vi "PlayWithSync.vi"() -> ()   [LabVIEW 2017]
uses:
  <vilib>/DAQmx/write.llb/DAQmx Write (Digital Wfm 1Chan NSamp).vi
  <vilib>/DAQmx/write.llb/DAQmx Write (Analog 1D Wfm NChan NSamp).vi
  <vilib>/DAQmx/create/channels.llb/DAQmx Create Channel (AO-Voltage-Basic).vi
  <vilib>/DAQmx/create/channels.llb/DAQmx Create Channel (DO-Digital Output).vi
  <vilib>/Waveform/DWDTOps.llb/DWDT Analog to Digital.vi
  <vilib>/DAQmx/configure/timing.llb/DAQmx Timing (Use Waveform).vi
  <vilib>/DAQmx/miscellaneous.llb/DAQmx Fill In Error Info.vi
  <vilib>/Waveform/DWDTOps.llb/DWDT Uncompress Digital.vi
panel:
  in  "Analog Input Sample Clock Source":tag="/Dev1/ao/SampleClock"
  in  "4k Hz Filter":bool=TRUE
  in  "Line(s)":tag="Dev1/port0/line0"
  in  "Physical Channels":tag="Dev1/ao0:1"
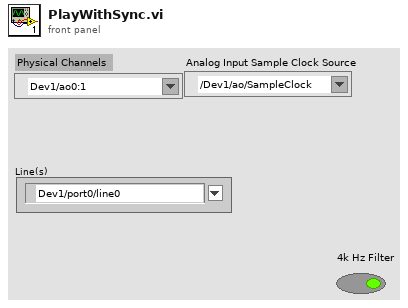
[diagram p1: front panel]
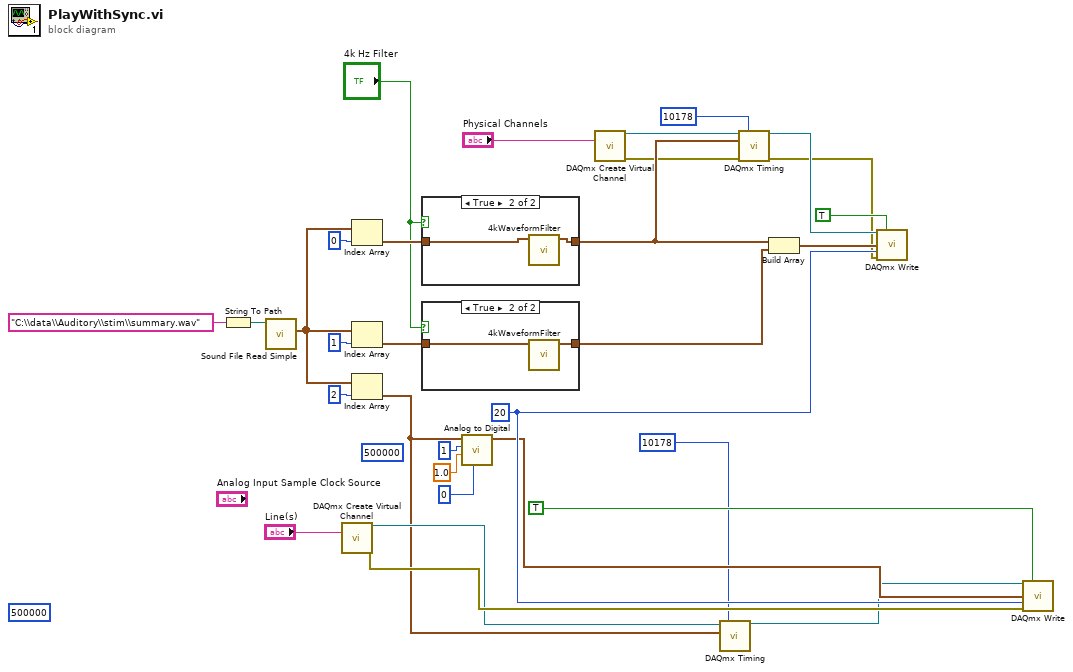
[diagram p0: block diagram]
diagram:
  (unwired) 500000
  (unwired) 500000
  w15 = 20
  n1 = String To Path(string="C:\\data\\Auditory\\stim\\summary.wav") -> (path=w31:path)
  n2 = call <vilib>:"Sound File Read Simple.vi"("path"=w31) -> ("data"=w25:waveform(dbl)[])  [unwired: 7 in, 3 out]
  n3 = call-poly <vilib>:"DAQmx Create Virtual Channel.vi"("lines"="Line(s)") -> ("task out"=w5:refnum<k21>, "error out"=w7:errorcluster)  [unwired: 13 in]
  n4 = Index Array(array=w25, index=0) -> (element=w18:waveform(dbl))
  n5 = Index Array(array=w25, index=1) -> (element=w19:waveform(dbl))
  n6 = Index Array(array=w25, index=2) -> (element=w2:waveform(dbl))
  n7 = case shown="True" "4k Hz Filter" {
    tunnel: w18 -> [w32 w34]
    tunnel: [w32 w33] -> w11
    frame False {
    }
    frame True {
      n8 = call "4kWaveformFilter.vi"("data"=w34) -> ("Waveform"=w33:waveform(dbl))  [unwired: 10 in]
    }
  }
  n9 = case shown="True" "4k Hz Filter" {
    tunnel: w19 -> [w35 w37]
    tunnel: [w35 w36] -> w14
    frame False {
    }
    frame True {
      n10 = call "4kWaveformFilter.vi"("data"=w37) -> ("Waveform"=w36:waveform(dbl))  [unwired: 10 in]
    }
  }
  n11 = call-poly <vilib>:"Analog to Digital.vi"("data format (offset binary)"=0, "full-scale range (pk-pk)"=1.0, "resolution (16 bit)"=1, "analog waveform"=w2) -> ("digital waveform"=w6:digitalwaveform)  [unwired: 4 in, 3 out]
  n12 = call-poly <vilib>:"DAQmx Create Virtual Channel.vi"("physical channels"="Physical Channels") -> ("task out"=w10:refnum<k21>, "error out"=w9:errorcluster)  [unwired: 13 in]
  n13 = call-poly <vilib>:"DAQmx Timing.vi"("task/channels in"=w5, "sample mode"=10178, "waveform"=w2) -> ("task out"=w4:refnum<k21>)  [unwired: 11 in, 1 out]
  n14 = call-poly <vilib>:"DAQmx Timing.vi"("task/channels in"=w10, "sample mode"=10178, "waveform"=w11, "error in"=w9) -> ("task out"=w16:refnum<k21>, "error out"=w8:errorcluster)  [unwired: 10 in]
  n15 = Build Array(w11, w14) -> (w13:waveform(dbl)[])
  n16 = call-poly <vilib>:"DAQmx Write.vi"("task/channels in"=w16, "auto start"=TRUE, "data"=w13, "timeout"=w15, "error in"=w8) -> ()  [unwired: 8 in, 3 out]
  n17 = call-poly <vilib>:"DAQmx Write.vi"("task/channels in"=w4, "auto start"=TRUE, "data"=w6, "timeout"=w15, "error in"=w7) -> ()  [unwired: 8 in, 3 out]
